vi "未命名 2.vi"() -> ()   [LabVIEW 2019]
panel:
  in  "节点-操作 2":T1={"ID"=0, "type"="dev", "flag"="", "name"="", "Act"={"Attribute"="dev", "Action"="", "Value"=0.0}} caption="簇 7" {"ID" format="%02x"}
  in  "节点-输出":T2(array[cluster])
  in  "节点-操作":T1={"ID"=0, "type"="dev", "flag"="", "name"="", "Act"={"Attribute"="dev", "Action"="", "Value"=0.0}} caption="簇 7" {"ID" format="%02x"}
  in  "数值":u8=1 min=1 max=6 step=1
  in  "节点组":T3(array[cluster]) {"ID" format="%02x"}
  in  "节点":T4={"ID"=0, "Attribute"="dev", "Action"="", "name"=""} {"ID" format="%02x"}
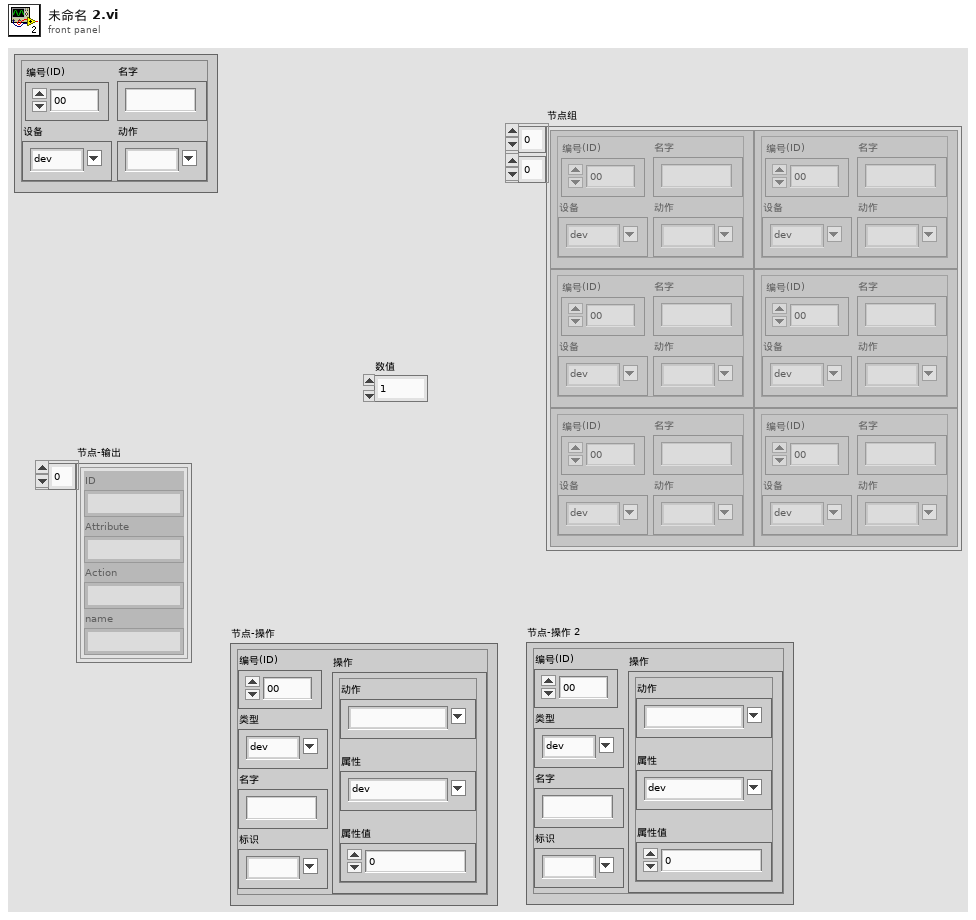
[diagram p1: front panel]
types:
  T1 = cluster{"ID":u8, "type":string, "flag":string, "name":string, "Act":cluster{"Attribute":string, "Action":string, "Value":dbl}}
  T2 = cluster{"ID":string, "Attribute":string, "Action":string, "name":string}[]
  T3 = cluster{"ID":u8, "Attribute":string, "Action":string, "name":string}[][]
  T4 = cluster{"ID":u8, "Attribute":string, "Action":string, "name":string}
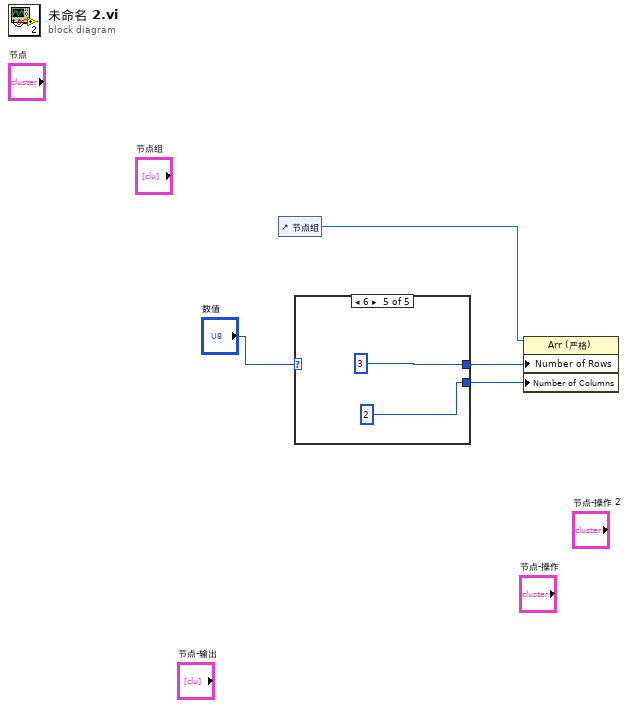
[diagram p0: block diagram]
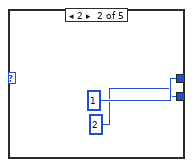
[diagram p3: hidden frame]
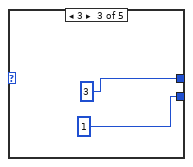
[diagram p4: hidden frame]
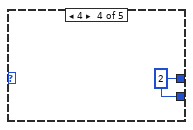
[diagram p5: hidden frame]
diagram:
  n1 = control-ref of="节点组"() -> (w4:refnum<vi>)
  n2 = case shown="6" "数值" {
    selector: "数值" -> [w5 _ _ _ _]
    tunnel: [w5 u8 1 ("数值") u8 3 ("数值") w10 u8 3 ("数值")] -> w2
    tunnel: [w5 u8 2 ("数值") u8 1 ("数值") w10 u8 2 ("数值")] -> w1
    frame 1, Default {
    }
    frame 2 {
    }
    frame 3 {
    }
    frame 4 {
      w10 = u8 2 ("数值")
    }
    frame 6 {
    }
  }
  n3 = property class="Arr (严格)"(reference=w4, "Number of Rows"=w2, "Number of Columns"=w1) -> ()  [unwired: 1 in, 2 out]
